vi "CanGrabberError.vi"(8 "error in (no error)":errorcluster) -> ()   [LabVIEW 2014]
uses:
  CanGrabberSetpoint.vi
panel:
  out "Time":u32
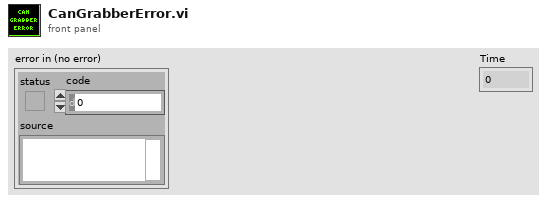
[diagram p1: front panel]
types:
  T1 = typedef "WPI_MotorControlDeviceRef.ctl" = cluster{"DeviceStatus":errorcluster, "Type":T2, "PWM":cluster{"Controller":T3, "PWM Channel":T4, "DeadBand":T5}, "CAN":cluster{"Device Number":u8, "Control Mode":T6, "Semaphore":T7, "Max Vout":dbl, "TalonSRX Control Mode":T8}, "Invert":bool, "TransformRef":T9, "InvTransformRef":T9}
  T2 = typedef "WPI_MotorControlType.ctl" = enum16{"PWM", "CAN", "CANTalonSRX"}
  T3 = typedef "FPGA_TypedefDigitalModule.ctl" = enum16{"Controller 1"}
  T4 = typedef "FPGA_DIOPWMChannel.ctl" = enum8{"PWM 0", "PWM 1", "PWM 2", "PWM 3", "PWM 4", "PWM 5", "PWM 6", "PWM 7", "PWM 8", "PWM 9", "PWM MXP 0", "PWM MXP 1", "PWM MXP 2", "PWM MXP 3", "PWM MXP 4", "PWM MXP 5", "PWM MXP 6", "PWM MXP 7", "PWM MXP 8", "PWM MXP 9", "Invalid"}
  T5 = typedef "WPI_PWMDeadband.ctl" = cluster{"Name":string, "maxPositivePwm":i32, "minPositivePwm":i32, "centerPwm":i32, "maxNegativePwm":i32, "minNegativePwm":i32, "angularRange":u16}
  T6 = typedef "WPI_CANJaguar_ControlMode.ctl" = enum8{"Percent VBus", "Current", "Speed", "Position", "Voltage"}
  T7 = typedef "Semaphore RefNum" = refnum<k1>
  T8 = typedef "WPI_CANTalonSRX_APIControlMode.ctl" = enum8{"Percent VBus", "Speed", "Position", "Slave", "Unchanged / Invalid"}
  T9 = typedef "WPI_PWMTransform_ConPane.ctl" = refnum<vi>
  T10 = typedef "WPI_CANTalonSRX_GlobalStatus.ctl" = cluster{"Applied Throttle":dbl, "Module Enabled":bool, "CAN Error":errorcluster, "Closed Loop Error":dbl, "Forward Limit Switch Closed":bool, "Reverse Limit Switch Closed":bool, "Sensor Position":dbl, "Sensor Velocity":dbl, "Current":dbl, "Sticky Fault - Over Temp":bool, "Sticky Fault - Under Voltage":bool, "Sticky Fault - Forward Limit":bool, "Sticky Fault - Reverse Limit":bool, "Sticky Fault - Forward Soft Limit":bool, "Sticky Fault - Reverse Soft Limit":bool, "Brake is Enabled":bool, "Encoder Position":dbl, "Encoder Velocity":dbl, "Encoder Index Count":dbl, "Encoder A Pin State":bool, "Encoder B Pin State":bool, "Encoder Index Pin State":bool, "Analog In":dbl, "Analog In Velocity":dbl, "Temperature (C)":dbl, "Battery Voltage":dbl}
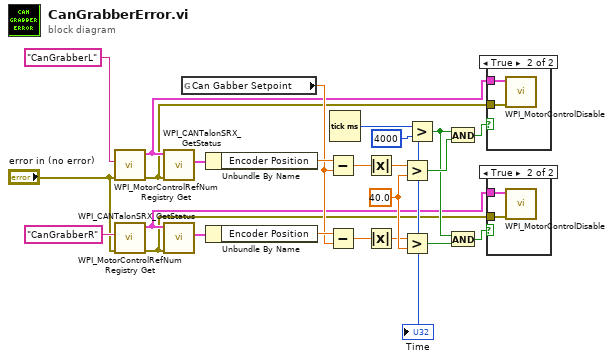
[diagram p0: block diagram]
diagram:
  w15 = 40.0 ("y")
  n1 = call <vilib>:"WPI_MotorControlRefNum Registry Get.vi"("error in (no error)"="error in (no error)", "refnum name"="CanGrabberL") -> ("error out"=w3:errorcluster, "MotorControlDevRef"=w4:T1)  [unwired: 8 in]
  n2 = call <vilib>:"WPI_MotorControlRefNum Registry Get.vi"("error in (no error)"="error in (no error)", "refnum name"="CanGrabberR") -> ("error out"=w1:errorcluster, "MotorControlDevRef"=w2:T1)  [unwired: 8 in]
  n3 = call <vilib>:"WPI_CANTalonSRX_GetStatus.vi"("error in (no error)"=w3, "CAN Talon SRX Ref"=w4) -> ("Talon SRX Status"=w22:T10)  [unwired: 7 in, 2 out]
  n4 = call <vilib>:"WPI_CANTalonSRX_GetStatus.vi"("error in (no error)"=w1, "CAN Talon SRX Ref"=w2) -> ("Talon SRX Status"=w21:T10)  [unwired: 7 in, 2 out]
  n5 = global read "CanGrabberSetpoint.vi" "Can Gabber Setpoint"() -> (w18:dbl)
  n6 = Unbundle By Name(w22) -> ("Encoder Position"=w20:dbl)
  n7 = Unbundle By Name(w21) -> ("Encoder Position"=w19:dbl)
  n8 = Subtract(x=w20, y=w18) -> (x-y=w16:dbl)
  n9 = Subtract(x=w19, y=w18) -> (x-y=w17:dbl)
  n10 = Tick Count (ms)() -> (millisecond timer value=w12:u32)
  "Time" <- w12
  n11 = Absolute Value(x=w16) -> (abs(x)=w14:dbl)
  n12 = Absolute Value(x=w17) -> (abs(x)=w13:dbl)
  n13 = Greater?(x=w14, y=w15) -> (0:w10:bool)
  n14 = Greater?(x=w13, y=w15) -> (0:w8:bool)
  n15 = Greater?(x=w12, y=u32 4000) -> (0:w7:bool)
  n16 = And(x=w7, y=w10) -> (x .and. y?=w6:bool)
  n17 = And(x=w7, y=w8) -> (x .and. y?=w5:bool)
  n18 = case shown="True" w6 {
    tunnel: w4 -> [_ w26]
    tunnel: w3 -> [_ w25]
    frame False {
    }
    frame True {
      n19 = call <vilib>:"WPI_MotorControlDisable.vi"("error in (no error)"=w25, "MotorControlDevRef"=w26) -> ()  [unwired: 8 in, 2 out]
    }
  }
  n20 = case shown="True" w5 {
    tunnel: w2 -> [_ w28]
    tunnel: w1 -> [_ w27]
    frame False {
    }
    frame True {
      n21 = call <vilib>:"WPI_MotorControlDisable.vi"("error in (no error)"=w27, "MotorControlDevRef"=w28) -> ()  [unwired: 8 in, 2 out]
    }
  }
